vi "Logger 2.vi"(8 "RAW NAPEDY 2":T1, 9 "ON/OFF LOG":bool, 11 "path":path) -> ()   [LabVIEW 2015]
panel:
  out "concatenated string":string
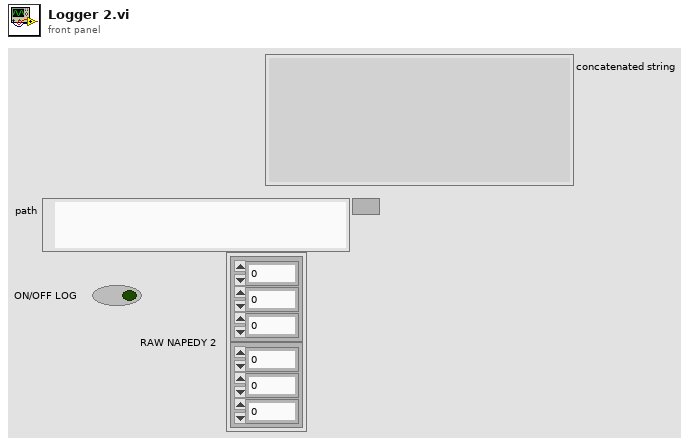
[diagram p1: front panel]
types:
  T1 = cluster{cluster{i16, i16, i16}, cluster{i16, i16, i16}}
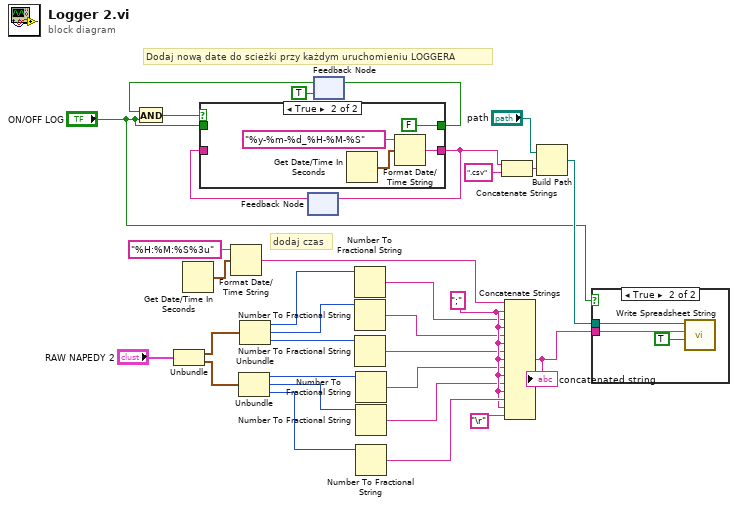
[diagram p0: block diagram]
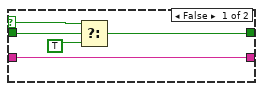
[diagram p3: hidden frame]
diagram:
  w31 = ";" ("delimiter (\\t)")
  # "dodaj czas"
  # "Dodaj nową date do scieżki przy każdym uruchomieniu LOGGERA"
  n1 = Unbundle("RAW NAPEDY 2") -> (w19:cluster{i16, i16, i16}, w15:cluster{i16, i16, i16})
  n2 = Get Date/Time In Seconds() -> (seconds since 1Jan1904=w25:timestamp)
  n3 = Format Date/Time String(time format string (%c)="%H:%M:%S%3u", seconds (now)=w25) -> (date/time string=w24:string)  [unwired: 1 in]
  n4 = Unbundle(w15) -> (w14:i16, w13:i16, w12:i16)
  n5 = Unbundle(w19) -> (w18:i16, w17:i16, w16:i16)
  n6 = feedback #1() -> (w6:string)  [unwired: 1 in]
  n7 = feedback #2(TRUE) -> (w3:bool)
  n8 = And(x=w3, y="ON/OFF LOG") -> (x .and. y?=w2:bool)
  n9 = case shown="True" w2 {
    selector: w2 -> [w33 _]
    tunnel: [w37 w39] -> w7
    tunnel: [w36 FALSE] -> w5
    tunnel: w6 -> [w37 _]
    tunnel: "ON/OFF LOG" -> [w34 _]
    frame False {
      n10 = Select(t=w33, s=w34, f=TRUE) -> (s? t:f=w36:bool)
    }
    frame True {
      n11 = Get Date/Time In Seconds() -> (seconds since 1Jan1904=w41:timestamp)
      n12 = Format Date/Time String(time format string (%c)="%y-%m-%d_%H-%M-%S", seconds (now)=w41) -> (date/time string=w39:string)  [unwired: 1 in]
    }
  }
  n13 = feedback-in #1(w7) -> ()
  n14 = feedback-in #2(w5) -> ()
  n15 = Number To Fractional String(number=w18) -> (F-format string=w23:string)  [unwired: 3 in]
  n16 = Number To Fractional String(number=w17) -> (F-format string=w22:string)  [unwired: 3 in]
  n17 = Number To Fractional String(number=w16) -> (F-format string=w21:string)  [unwired: 3 in]
  n18 = Number To Fractional String(number=w14) -> (F-format string=w29:string)  [unwired: 3 in]
  n19 = Number To Fractional String(number=w13) -> (F-format string=w30:string)  [unwired: 3 in]
  n20 = Number To Fractional String(number=w12) -> (F-format string=w32:string)  [unwired: 3 in]
  n21 = Concatenate Strings(w7, ".csv" ("string")) -> (w11:string)
  n22 = Concatenate Strings(w24, w31, w23, w31, w22, w31, w21, w31, w29, w31, w30, w31, w32, w31, "\r") -> (w27:string)
  "concatenated string" <- w27
  n23 = Build Path(base path="path", name or relative path=w11) -> (appended path=w8:path)
  n24 = case shown="True" "ON/OFF LOG" {
    tunnel: w27 -> [_ w44]
    tunnel: w8 -> [_ w42]
    frame False {
    }
    frame True {
      n25 = call <vilib>:"Write Spreadsheet String.vi"("append to file? (new file:F)"=TRUE, "spreadsheet string"=w44, "file path (dialog if empty)"=w42) -> ()  [unwired: 7 in, 2 out]
    }
  }
